vi "Actuators Get Moving Channel.vi"(0 "Notifier Name":string, 7 "Channel":i32, 11 "Error In":errorcluster) -> (4 "Notifier Name Out":string, 8 "Moving":bool, 15 "Error Out":errorcluster)   [LabVIEW 2020]
uses:
  Actuators Controls/Actuators Note Type.ctl
  Actuators Controls/Actuators Actions.ctl
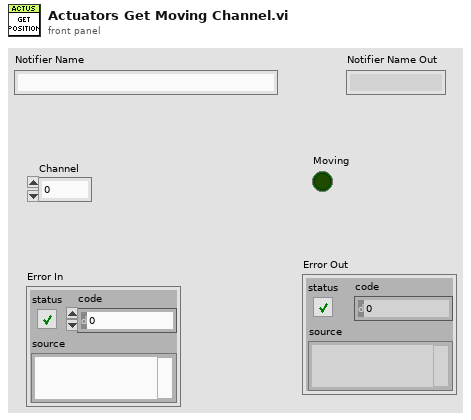
[diagram p1: front panel]
types:
  T1 = typedef "Actuators Note Type.ctl" = cluster{"Actions":T2, "Cmd Received ":bool, "Setpoint":dbl[], "Position":dbl[], "Channel":i32[], "Jog Step":dbl[], "Velocity":dbl[], "Acceleration":dbl[], "Status Bits":u32[], "Moving":bool[]}
  T2 = typedef "Actuators Actions.ctl" = enum16{"Nothing", "Get Position", "Get Acceleration", "Get Velocity", "Get Jog Step", "Set Acceleration", "Set Velocity", "Set Jog Step", "Move Absolute", "Move Relative", "Jog Forward", "Jog Reverse", "Set Moving", "Halt", "Quit"}
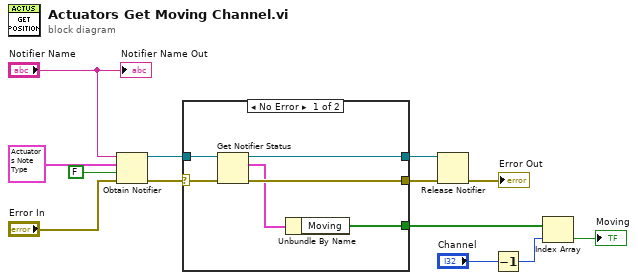
[diagram p0: block diagram]
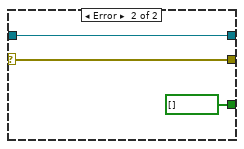
[diagram p2: hidden frame]
diagram:
  n1 = Obtain Notifier(name (unnamed)="Notifier Name", notification data type=T1 {"Actions"=enum."Nothing", "Cmd Received "=FALSE, "Setpoint"=[], "Position"=[], "Channel"=[], "Jog Step"=[], "Velocity"=[], "Acceleration"=[], "Status Bits"=[], "Moving"=[]} ("Actuators Note"), create if not found? (T)=FALSE, error in (no error)="Error In") -> (notifier out=w9:refnum<notifier>, error out=w12:errorcluster)  [unwired: 1 out]
  n2 = case shown="No Error" w12 {
    selector: w12 -> [w18 w21]
    tunnel: w9 -> [w19 w22]
    tunnel: [w17 w22] -> w8
    tunnel: [w16 w21] -> w7
    tunnel: [w14 bool[] [] ("Moving")] -> w4
    frame No Error {
      n3 = Get Notifier Status(notifier=w19, error in (no error)=w18) -> (notifier out=w17:refnum<notifier>, current notification=w15:T1, error out=w16:errorcluster)  [unwired: 2 out]
      n4 = Unbundle By Name(w15) -> ("Moving"=w14:bool[])
    }
    frame Error {
    }
  }
  n5 = Release Notifier(notifier=w8, error in (no error)=w7) -> (error out=→"Error Out":errorcluster)  [unwired: 1 in, 2 out]
  n6 = Decrement(x="Channel") -> (x-1=w2:i32)
  n7 = Index Array(array=w4, index=w2) -> (element=→"Moving":bool)
  "Notifier Name Out" <- "Notifier Name"
